vi "6-2.vi"() -> ()   [LabVIEW 2022 SP3, in "AoC22.lvlib"]
uses:
  AoC22.lvlib
panel:
  out "Numeric":i32
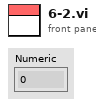
[diagram p1: front panel]
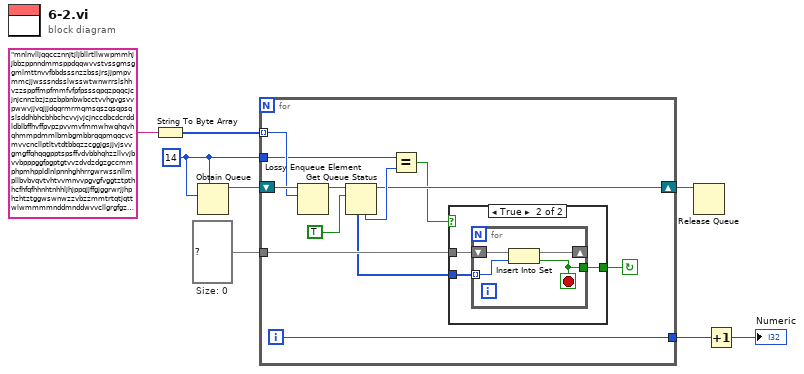
[diagram p0: block diagram]
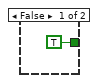
[diagram p2: hidden frame]
diagram:
  w4 = set{i32} {}  # Size: 0
  w1 = 14 ("max queue size (-1, unlimited)")
  n1 = String To Byte Array(string="mnlnvlljqqccznnjtjljbllrtllwwpmmhjjbbzppnndmmsppdqqwvvstvssgmsggmlmttnvvfbbdsssnzzbssjrsjjpmpvmmcjjwsssndsslwsswtwnwrrslshhvzzsppffmpfmmfvfpfpsssqpqzpqqcjcjnjcnnzbzjzpzbpbnbwbcctvvhgvgsvvpwwvjjvqjjjdqqrmrmqmsqszqsqpsqslsddhbhcbhbchcvvjvjcjnccdbcdcrddldblbffhvffpvpzpvvmvfmmwhwqhqvhqhmmpdmmlbmbgmbbrqqpmqqcvcmvvcncllptltvtdtbbqzzcggjgsjjvjsvvgmgffqhqqgpptspsffvdvbbhqhzzllvvjbvvbpppggfpgptgtvvzdvdzdgzgccmmphpmhppldlnlpnnhghhrrgwrwssnllmpllbvbvqvtvhtvvmnvvpgvgfvggtztpthhcfhfqfhhnhtnhhljhjppqjjffgjggrwrjjhphzhtztggwswnwzzvbzzmmtrtqtjqttwlwmmmmnddmnddwvvcllgrgfgzznwnsswjjhwwspsbbvzzqvzvbvcvmmtltnlnfn...") -> (unsigned byte array=w5:u8[])
  n2 = Obtain Queue(max queue size (-1, unlimited)=w1, element data type=w1) -> (queue out=w3:refnum<queue>)  [unwired: 3 in, 2 out]
  n3 = for {
    tunnel: w5 -> [w18] mode=indexing
    tunnel: [w20] -> w7
    tunnel: w4 -> [w11]
    shift-right: [w13] -> w2
    shift-left: w3 -> [w19]
    tunnel: w1 -> [w15]
    i -> [w20]
    stop <- w9 continue-if-true
    n4 = Lossy Enqueue Element(queue=w19, element=w18) -> (queue out=w17:refnum<queue>)  [unwired: 1 in, 3 out]
    n5 = Get Queue Status(queue=w17, return elements? (F)=TRUE) -> (queue out=w13:refnum<queue>, # elements in queue=w14:i32, elements=w10:i32[])  [unwired: 1 in, 5 out]
    n6 = Equal?(x=w15, y=w14) -> (x = y?=w12:bool)
    n7 = case shown="True" w12 {
      tunnel: w11 -> [_ w24]
      tunnel: w10 -> [_ w23]
      tunnel: [TRUE ("already included?") w22] -> w9
      frame False {
      }
      frame True {
        n8 = for {
          tunnel: w23 -> [w27] mode=indexing
          shift-right: [w26] -> _
          shift-left: w24 -> [w28]
          tunnel: [w25] -> w22
          stop <- w25 stop-if-true
          n9 = Insert Into Set(10:w27, 11:w28) -> (2:w25:bool, 3:w26:set{i32})
        }
      }
    }
  }
  n10 = Release Queue(queue=w2) -> ()  [unwired: 2 in, 3 out]
  n11 = Increment(x=w7) -> (x+1=→"Numeric":i32)
